vi "Convert IV Data.vi"(4 "Voltmeter after preamp":bool=TRUE, 5 "Current range":dbl=0.001 format="%#_6pA", 6 "Preamp gain":dbl=5.0 format="%#_6f", 7 "Lock-in Vout":dbl=0.02 format="%#_6pV", 8 "V index":i32, 9 "I-V index":i32=2, 10 "Data in":waveform(dbl)[](array[waveform]), 11 "Measurement technique":T1(ring)=enum."Lock-in dV/dI") -> (2 "Data out":waveform(dbl)[](array[waveform]))   [LabVIEW 2021]
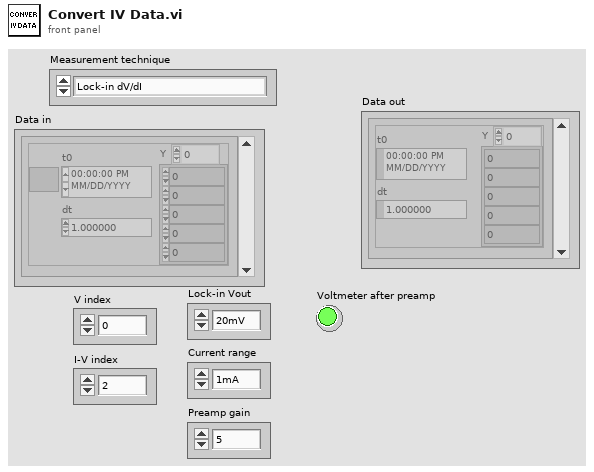
[diagram p1: front panel]
types:
  T1 = enum16{"", "Lock-in dV/dI", "Keithley 6221/2182 "}
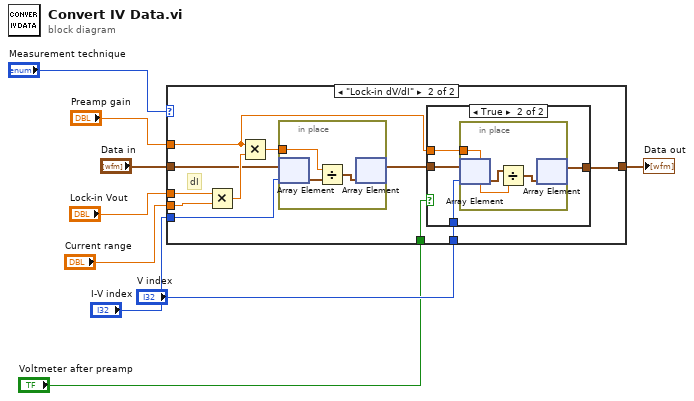
[diagram p0: block diagram]
diagram:
  n1 = case shown="\"Lock-in dV/dI\"" "Measurement technique" {
    tunnel: "Data in" -> [w10 w17]
    tunnel: "I-V index" -> [_ w16]
    tunnel: "Lock-in Vout" -> [_ w21]
    tunnel: "Current range" -> [_ w20]
    tunnel: "Preamp gain" -> [_ w12]
    tunnel: [w10 w14] -> w3
    tunnel: "V index" -> [_ w13]
    tunnel: "Voltmeter after preamp" -> [_ w11]
    frame "", Default {
    }
    frame "Lock-in dV/dI" {
      # "dI"
      n2 = Multiply(x=w21, y=w20) -> (x*y=w19:dbl)
      n3 = Multiply(x=w12, y=w19) -> (x*y=w18:dbl)
      n4 = in-place {
        in-place-border: w18 -> [w32]
        n5 = in-place-array #1(w17, w16) -> (w31:waveform(dbl))
        n6 = Divide(x=w32, y=w31) -> (x/y=w30:waveform(dbl))
        n7 = in-place-array #1(w30) -> (w15:waveform(dbl)[])  [unwired: 1 out]
      }
      n8 = case shown="True" w11 {
        tunnel: w15 -> [w22 w26]
        tunnel: [w22 w25] -> w14
        tunnel: w13 -> [_ w24]
        tunnel: w12 -> [_ w23]
        frame False {
        }
        frame True {
          n9 = in-place {
            in-place-border: w23 -> [w27]
            n10 = in-place-array #2(w26, w24) -> (w28:waveform(dbl))
            n11 = Divide(x=w28, y=w27) -> (x/y=w29:waveform(dbl))
            n12 = in-place-array #2(w29) -> (w25:waveform(dbl)[])  [unwired: 1 out]
          }
        }
      }
    }
  }
  "Data out" <- w3
